vi "Module Cleanup.vi"(8 "error in (no error)":errorcluster, 11 "System Config Server in":refnum<class "System Config Server.lvclass">) -> (0 "error out":errorcluster, 3 "System Config Server out":refnum<class "System Config Server.lvclass">)   [LabVIEW 2020, in "Volatus.lvlib" / "System Config Server.lvclass"]
uses:
  System Config Server.lvclass
  System Config Server.lvclass/System Config Server.ctl
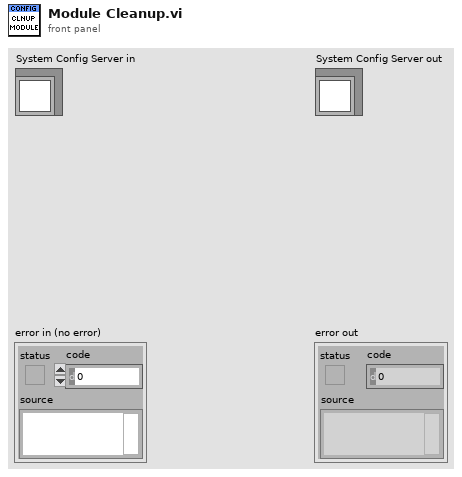
[diagram p1: front panel]
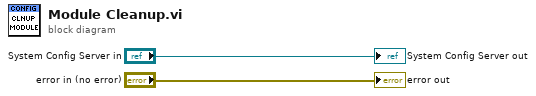
[diagram p0: block diagram]
diagram:
  "error out" <- "error in (no error)"
  "System Config Server out" <- "System Config Server in"
